vi "DDS_client.vi"() -> ()   [LabVIEW 2012]
uses:
  <userlib>/LabRAD/internal/Build Packet SubVIs/Build Packet by Name.vi
  <userlib>/LabRAD/internal/Simple Request SubVIs/Simple Request by Name.vi
panel:
  in  "DDS":cluster{string, dbl, dbl}={"866DP", 80.0, -5.0} {"?" min=80.0 max=100.0 step=0.001; "?" min=-63.0 max=-5.0 step=0.001}
  in  "update":bool
  out "client ID":u32
  out "welcome message":string
  in  "manager":T1={"address"="localhost", "port"=7682, "password"=""}
  # "Name"
  # "Freq (MHz)"
  # "Amp (dBm)"
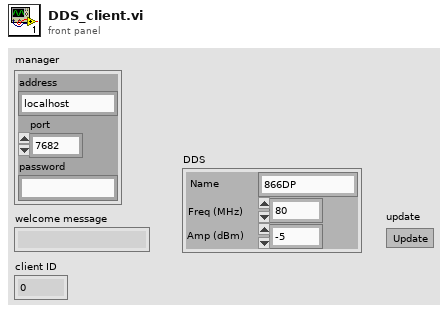
[diagram p1: front panel]
types:
  T1 = cluster{"address":string, "port":u16, "password":string}
  T2 = cluster{"Setting":cluster{"ID":u32, "Name":string}, "Type Tag":string, "Data":string}[]
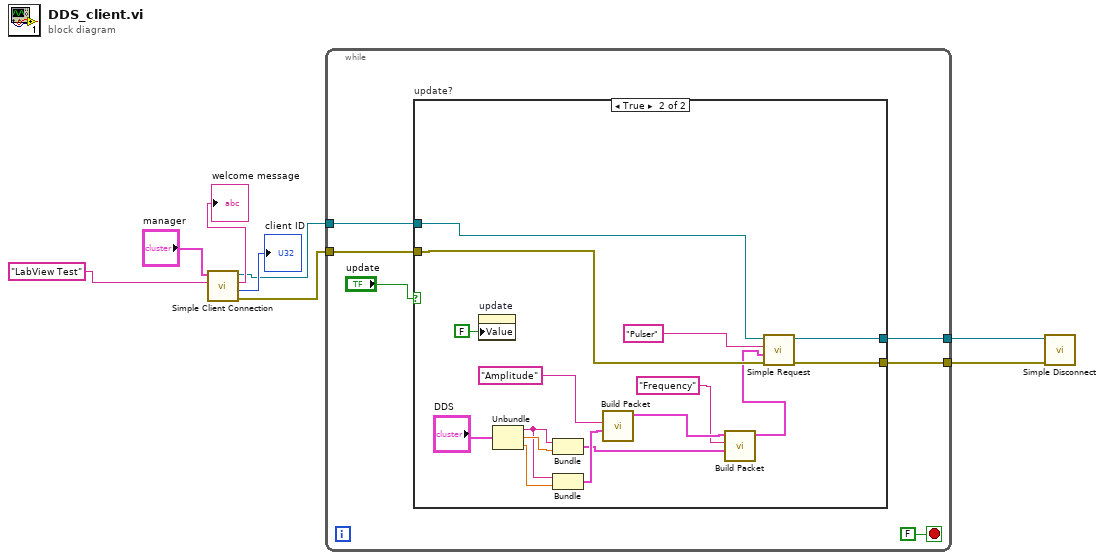
[diagram p0: block diagram]
diagram:
  n1 = call <userlib>:"Simple Client Connection.vi"("connection name (LabVIEW Client)"="LabView Test", "manager"="manager") -> ("error out"=w4:errorcluster, "client ID"=→"client ID":u32, "welcome message"=→"welcome message":string, "connection ID out"=w3:refnum<k5>)  [unwired: 2 in]
  n2 = while {
    tunnel: w4 -> [w12]
    tunnel: w3 -> [w11]
    tunnel: [w10] -> w2
    tunnel: [w9] -> w1
    stop <- FALSE stop-if-true
    n3 = case "update?" shown="True" "update" {
      tunnel: w12 -> [w15 w28]
      tunnel: w11 -> [w16 w29]
      tunnel: [w16 w27] -> w10
      tunnel: [w15 w26] -> w9
      frame False {
      }
      frame True {
        n4 = property on="update" class="Bool (strict)"("Value"=FALSE ("update")) -> ()  [unwired: 2 in, 2 out]
        n5 = Unbundle("DDS") -> (w23:string, w24:dbl, w22:dbl)
        n6 = Bundle(w23, w24) -> (w18:cluster{string, dbl})  [unwired: 1 in]
        n7 = Bundle(w23, w22) -> (w21:cluster{string, dbl})  [unwired: 1 in]
        n8 = call-poly <userlib>:"Build Packet.vi"("data (empty)"=w21, "setting"="Amplitude") -> ("appended records"=w20:T2)  [unwired: 6 in, 2 out]
        n9 = call-poly <userlib>:"Build Packet.vi"("data (empty)"=w18, "setting"="Frequency", "records (empty)"=w20) -> ("appended records"=w19:T2)  [unwired: 5 in, 2 out]
        n10 = call-poly <userlib>:"Simple Request.vi"("error in (no error)"=w28, "records in (empty)"=w19, "target (Manager)"="Pulser", "connection ID"=w29) -> ("error out"=w26:errorcluster, "connection ID out"=w27:refnum<k5>)  [unwired: 2 in, 2 out]
      }
    }
  }
  n11 = call <userlib>:"Simple Disconnect.vi"("error in (no error)"=w1, "connection ID"=w2) -> ()  [unwired: 5 in, 1 out]
